vi "Status Heater.vi"(8 "error in (no error)":errorcluster, 10 "Loop":u16(ring)=1 items=["Loop 1", "Loop 2"], 11 "VISA resource name":refnum<visa-resource-name>="GPIB0::14::INSTR") -> (0 "error out":errorcluster, 1 "Heater Range":enum16{"Off", "1", "2", "3", "4", "5"}(ring), 3 "VISA resource name out":refnum<visa-resource-name>)   [LabVIEW 2019, in "Lake Shore Cryotronics 340.lvlib"]
uses:
  Lake Shore Cryotronics 340.lvlib
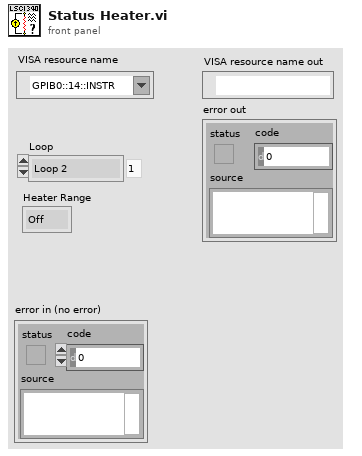
[diagram p1: front panel]
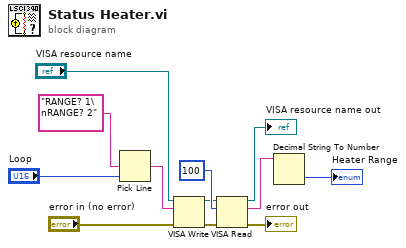
[diagram p0: block diagram]
diagram:
  n1 = Pick Line(multi-line string="RANGE? 1\nRANGE? 2", line index="Loop") -> (output string=w6:string)  [unwired: 1 in]
  n2 = VISA Write(VISA resource name="VISA resource name", write buffer=w6, error in (no error)="error in (no error)") -> (VISA resource name out=w8:refnum<visa-resource-name>, error out=w7:errorcluster)  [unwired: 1 out]
  n3 = VISA Read(VISA resource name=w8, byte count=100, error in (no error)=w7) -> (VISA resource name out=→"VISA resource name out":refnum<visa-resource-name>, read buffer=w3:string, error out=→"error out":errorcluster)  [unwired: 1 out]
  n4 = Decimal String To Number(string=w3) -> (number=→"Heater Range":i32)  [unwired: 2 in, 1 out]
